vi "Command_SetRobotPose.vi"(7 "Parameters":dbl[](array[numeric]), 11 "Startup":bool) -> (4 "Completed":bool, 15 "Reinit":bool)   [LabVIEW 2019]
uses:
  Auto Utilities/Command_Execution_State.ctl
  Globals/Drive_Globals.vi
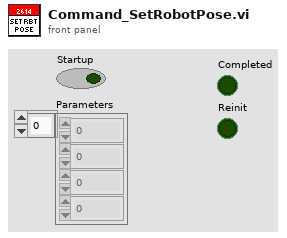
[diagram p1: front panel]
types:
  T1 = typedef "Command_Execution_State.ctl" = enum16{"Initialize", "Execute", "Finish"}
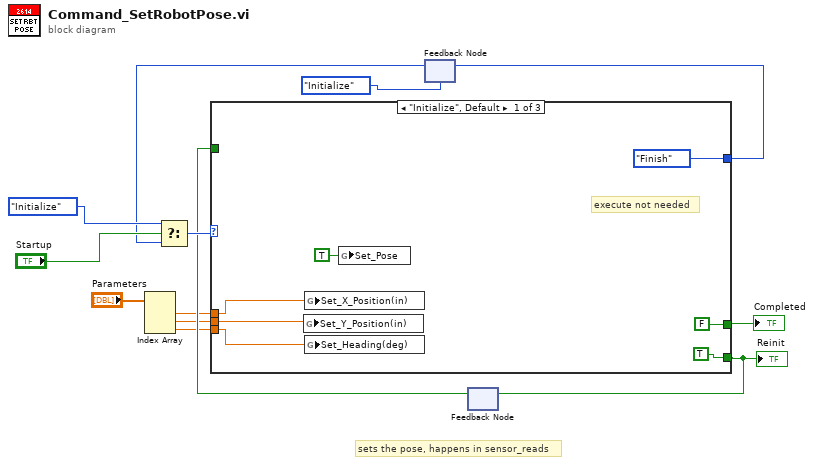
[diagram p0: block diagram]
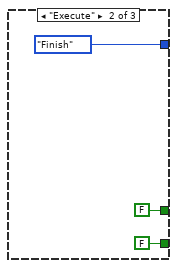
[diagram p2: hidden frame]
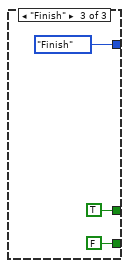
[diagram p3: hidden frame]
diagram:
  # "sets the pose, happens in sensor_reads"
  n1 = Index Array(array="Parameters") -> (element #1=w3:dbl, element #2=w2:dbl, element #3=w1:dbl)  [unwired: 3 in]
  n2 = feedback #1(Command_Execution_State."Initialize") -> (w9:T1)
  n3 = Select(t=Command_Execution_State."Initialize", s="Startup", f=w9) -> (s? t:f=w11:T1)
  n4 = feedback #2() -> (w5:bool)  [unwired: 1 in]
  n5 = case shown="\"Initialize\", Default" w11 {
    tunnel: [Command_Execution_State."Finish" Command_Execution_State."Finish" Command_Execution_State."Finish"] -> w10
    tunnel: [FALSE ("Reinit") FALSE ("Reinit") TRUE ("Reinit")] -> w7
    tunnel: [TRUE ("Reinit") FALSE ("Reinit") FALSE ("Reinit")] -> w6
    tunnel: w5 -> [_ _ _]
    tunnel: w3 -> [w16 _ _]
    tunnel: w2 -> [w15 _ _]
    tunnel: w1 -> [w14 _ _]
    frame "Initialize", Default {
      # "execute not needed"
      n6 = global write "Drive_Globals.vi" "Set_Y_Position(in)"(w15) -> ()
      n7 = global write "Drive_Globals.vi" "Set_X_Position(in)"(w16) -> ()
      n8 = global write "Drive_Globals.vi" "Set_Heading(deg)"(w14) -> ()
      n9 = global write "Drive_Globals.vi" "Set_Pose"(TRUE ("Set_Pose")) -> ()
    }
    frame "Execute" {
    }
    frame "Finish" {
    }
  }
  "Reinit" <- w6
  "Completed" <- w7
  n10 = feedback-in #1(w10) -> ()
  n11 = feedback-in #2(w6) -> ()
